vi "get last banking transaction.vi"(8 "error in (no error)":errorcluster, 11 "Database in":refnum<class "Database.lvclass">) -> (0 "error out":errorcluster, 3 "Database out":refnum<class "Database.lvclass">)   [LabVIEW 2018, in "Database.lvclass"]
uses:
  Database.lvclass
  Banking Record/Banking Record.lvclass
panel:
  out "Last Banking Transaction":refnum<class "Banking Record.lvclass">
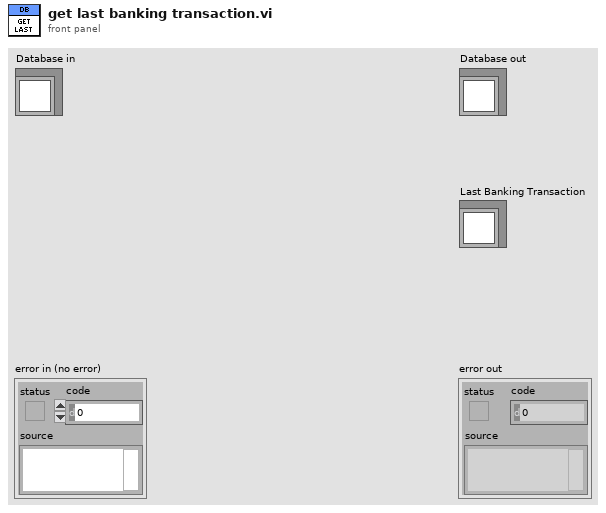
[diagram p1: front panel]
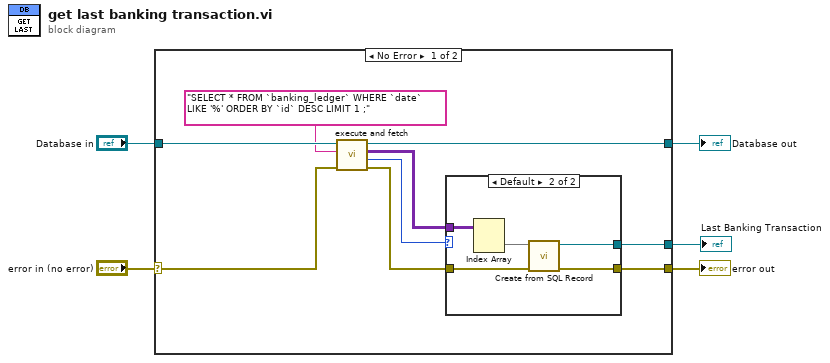
[diagram p0: block diagram]
diagram:
  n1 = case shown="No Error" "error in (no error)" {
    selector: "error in (no error)" -> [w12 w22]
    tunnel: [w9 w22] -> w4
    tunnel: [w13 w21] -> w2
    tunnel: "Database in" -> [w14 w21]
    tunnel: [w6 _] -> w1
    frame No Error {
      n2 = call "execute and fetch.vi"("error in (no error)"=w12, "SQL query"="SELECT * FROM `banking_ledger` WHERE `date` LIKE '%' ORDER BY `id` DESC LIMIT 1 ;", "Database in"=w14) -> ("error out"=w10:errorcluster, "No records"=w7:i32, "recordset data"=w8:variant[][], "Database out"=w13:refnum<class "Database.lvclass">)  [unwired: 5 in]
      n3 = case shown="Default" w7 {
        tunnel: w10 -> [w15 w18]
        tunnel: [w15 w17] -> w9
        tunnel: w8 -> [_ w20]
        tunnel: [_ w16] -> w6
        frame 0 {
        }
        frame Default {
          n4 = Index Array(array=w20) -> (element=w19:variant[])  [unwired: 2 in]
          n5 = call "Create from SQL Record.vi"("error in (no error)"=w18, "MySQL Record"=w19) -> ("error out"=w17:errorcluster, "Banking Record"=w16:refnum<class "Banking Record.lvclass">)  [unwired: 8 in]
        }
      }
    }
    frame Error {
    }
  }
  "error out" <- w4
  "Database out" <- w2
  "Last Banking Transaction" <- w1
